vi "Reinitial Parameter After Test.vi"(8 "error in (no error)":errorcluster, 11 "main ref":T1) -> (0 "error out":errorcluster)   [LabVIEW 2025]
uses:
  controls/LAB-IQ UI Data.ctl
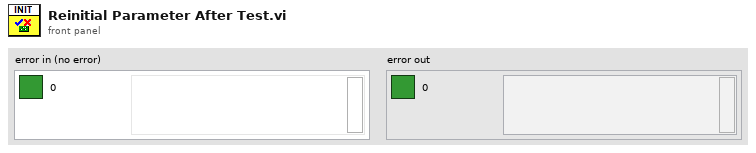
[diagram p1: front panel]
types:
  T1 = typedef "LAB-IQ UI Data.ctl" = cluster{"Main Home Screen":cluster{"GUI":refnum<vi>, "Platform Settings":refnum<vi>, "Configure":refnum<vi>, "Home":refnum<vi>, "EXIT":refnum<vi>, "service 2":refnum<vi>, "MainPage":refnum<vi>, "Analysis":refnum<vi>}, "Platform Settings":cluster{"mm/s  Surge":refnum<vi>, "Update Surge Speed":refnum<vi>, "Drive Error":refnum<vi>, "Disable Axis Jog Soft Limits":refnum<vi>, "mm/s  Sway":refnum<vi>, "Sway and Surge COM Status":refnum<vi>, "Heave COM Status":refnum<vi>, "Enable Platform":refnum<vi>, "Surge Forward Main":refnum<vi>, "Sway Right Main":refnum<vi>, "Sway Left Main":refnum<vi>, "Heave Down Main":refnum<vi>, "Heave Up main":refnum<vi>, "Update Sway Speed":refnum<vi>, "Update Heave Speed":refnum<vi>, "mm/s Heave":refnum<vi>, "mm/sec":refnum<vi>, "mm":refnum<vi>, "Surge Backward Main":refnum<vi>}, "Analysis Screen":cluster{"Analysis Home":refnum<vi>, "Surface Analysis":refnum<vi>, "Imaging":refnum<vi>, "Image Analysis":refnum<vi>, "Post Analysis":refnum<vi>}, "Config Screen":cluster{"Select Load Head":refnum<vi>, "Notes :":refnum<vi>, "FILE":refnum<vi>, "Sample ID :":refnum<vi>, "Operator ID :":refnum<vi>, "Operator Name :":refnum<vi>, "Auto":refnum<vi>}, "Motion Module":cluster{"zNL":refnum<vi>, "NL disp":refnum<vi>, "Rotary Tab":refnum<vi>, "Motion Direction:  3":refnum<vi>, "E.Velocity 2":refnum<vi>, "e.v/ssr 2":refnum<vi>, "Enter Fixed E.Velocity 2":refnum<vi>, "Enter Final SRR 2":refnum<vi>, "Enter initial SRR 2":refnum<vi>, "Enter Fixed SRR 2":refnum<vi>, "Enter the Final E.Velocity (m/s) 2":refnum<vi>, "Enter initial E.Velocity (m/s) 2":refnum<vi>, "Final Speed (RPM) 3":refnum<vi>, "Initial Speed (RPM) 2":refnum<vi>, "Enter the Final Velocity (m/s) 3":refnum<vi>, "Enter initial Velocity (m/s)  3":refnum<vi>, "Ramp Up 2":refnum<vi>, "TEST SELECTION":refnum<vi>, "SPEED SELECTION : ":refnum<vi>, "Angular Oscillation Set":refnum<vi>, "Traction":refnum<vi>, "Step Speed":refnum<vi>, "StepTable For Load-Speed":refnum<vi>, "StepTable For Speed":refnum<vi>, "Surge Forward MM":refnum<vi>, "Surge Backward MM":refnum<vi>, "M3 Image":refnum<vi>, "String 39":refnum<vi>, "Sway Left MM":refnum<vi>, "Sway Right MM":refnum<vi>, "Disable Axis Jog Soft Limits":refnum<vi>, "mm":refnum<vi>, "Heave Down MM":refnum<vi>, "Heave Up MM":refnum<vi>, "Wear Track Diameter (mm)":refnum<vi>, "Set WTD":refnum<vi>, "HomeScratch":refnum<vi>, "HomeRot":refnum<vi>, "PlaceModule":refnum<vi>, "Enter the Angle (Deg)":refnum<vi>, "Enter the Frequency (Hz)":refnum<vi>, "Motion Mode:":refnum<vi>, "LR Sway":refnum<vi>, "Rot Hor":refnum<vi>, "Scratch":refnum<vi>, "LR Cam":refnum<vi>, "MMBack":refnum<vi>, "MMNext":refnum<vi>, "Rot Ver":refnum<vi>, "Rotary Module Selection":refnum<vi>, "calculate rotary":refnum<vi>, "SPEED SELECTION : rotary":refnum<vi>, "Import 2":refnum<vi>, "Save 2":refnum<vi>, "File Path :  2":refnum<vi>, "String 45":refnum<vi>, "StepTable For Speed 3":refnum<vi>, "Enter the Speed(mm/sec)":refnum<vi>, "Enter the Speed(RPM)":refnum<vi>, "Enter Scratch Speed (mm/s):":refnum<vi>, "SwaySpeed Set":refnum<vi>, "Scartch Offset":refnum<vi>, "Motion type:":refnum<vi>, "HomeScratch 2":refnum<vi>, "Enter Scratch length (mm):":refnum<vi>, "Wear Track Diameter":refnum<vi>, "Rotary Speed Exced":refnum<vi>, "Scratch Mode":refnum<vi>, "No of Scratch":refnum<vi>}, "Environmental control":cluster{"Humidity  Status  3":refnum<vi>, "Low Temp  Status  2":refnum<vi>, "TK4 status 2":refnum<vi>, "Stage Temperature":refnum<vi>, "Sample Temperature":refnum<vi>, "Humidity (Amb)":refnum<vi>, "Clear List":refnum<vi>, "Add to list":refnum<vi>, "Wear":refnum<vi>, "Vibration":refnum<vi>, "Humidity (Chamber)":refnum<vi>, "Temperature (Chamber)":refnum<vi>, "ECR ":refnum<vi>, "Temperature (Amb)":refnum<vi>, "Microphone":refnum<vi>, "Acoustic Emission 3":refnum<vi>, "SNext":refnum<vi>, "APBack":refnum<vi>, "Enter the Temperature (°C):":refnum<vi>, "Enter the Stage \nTemperature (°C):":refnum<vi>, "Enter the Humidity (%Rh):":refnum<vi>, "Low Temp":refnum<vi>, "High Temp":refnum<vi>, "Humidity":refnum<vi>, "Sensors Picked":refnum<vi>}, "About Screen":cluster{"Password":refnum<vi>, "Home Service":refnum<vi>, "Advanced Setting":refnum<vi>, "About Tab":refnum<vi>, "ECR Port:":refnum<vi>, "Ramp Port:":refnum<vi>, "Installation/Replacement completed":refnum<vi>, "Loahead":refnum<vi>, "Heave and Surge COM Port:":refnum<vi>, "Sway COM Port:":refnum<vi>, "Temp Modbus:":refnum<vi>, "Humidity Port:":refnum<vi>, "Edit Gain Constants":refnum<vi>, "Save Gain Constants":refnum<vi>}, "Main Screen":cluster{"Main Screen Tab":refnum<vi>, "Angle and Frequency":refnum<vi>, "Stroke (mm)":refnum<vi>, "Angle (Deg)":refnum<vi>, "Main Speed Tab":refnum<vi>, "MTM MOTOR DISPLAY":refnum<vi>, "Disc Speed (m/sec)":refnum<vi>, "Ball Speed (m/sec)":refnum<vi>, "Disc Speed (RPM)":refnum<vi>, "Ball Speed (RPM)":refnum<vi>, "SPEED TAB":refnum<vi>, "Speed (m/sec)":refnum<vi>, "Set Speed (m/sec)":refnum<vi>, "Speed (RPM)":refnum<vi>, "Set Speed":refnum<vi>, "Time Tab":refnum<vi>, "Time ( HH:MM:SS ) 2":refnum<vi>, "Test Duration":refnum<vi>, "Test Duration 4":refnum<vi>, "TEST CYCLE":refnum<vi>, "TOTAL CYCLES":refnum<vi>, "Set Load (N)":refnum<vi>, "Temp Tabs":refnum<vi>, "Heater":refnum<vi>, "TK4 status":refnum<vi>, "ChamberTemp":refnum<vi>, "SetTmp":refnum<vi>, "Controller  Status":refnum<vi>, "ChamberTemp 2":refnum<vi>, "SetTmp 2":refnum<vi>, "Controller  Status 2":refnum<vi>, "ChamberTemp 3":refnum<vi>, "SetTmp 3":refnum<vi>, "Cooling":refnum<vi>, "Load Communication":refnum<vi>, "Ambient \nTemperature":refnum<vi>, "HumCOMStatus":refnum<vi>, "Ambient\n Humidity":refnum<vi>, "Freq (Hz)":refnum<vi>, "Load En":refnum<vi>, "NLt":refnum<vi>, "zNL 2":refnum<vi>, "Humidity On":refnum<vi>, "humidity disp":refnum<vi>, "Set Humidity":refnum<vi>, "NL disp 2":refnum<vi>, "Humidity On 2":refnum<vi>, "humidity disp 2":refnum<vi>, "Set Humidity 2":refnum<vi>, "NL disp 3":refnum<vi>, "AppLoadSeq scratch":refnum<vi>, "Stop Scratch":refnum<vi>, "ClrLog":refnum<vi>, "Trip Log":refnum<vi>, "STOP":refnum<vi>, "Start Test":refnum<vi>, "Test status":refnum<vi>, "AR Led":refnum<vi>, "Data":refnum<vi>, "Health":refnum<vi>, "Sway COM Status":refnum<vi>, "Heave COM Status":refnum<vi>, "Grp Tab":refnum<vi>, "Sub Graph":refnum<vi>, "SD (mm)":refnum<vi>, "Siliding distance Reset Graph":refnum<vi>, "SDGp":refnum<vi>, "Humidity Reset Graph":refnum<vi>, "HumrGp":refnum<vi>, "Acoustic Emission (mV)":refnum<vi>, "Aqucostic Reset Graph":refnum<vi>, "gACQUOS":refnum<vi>, "ECR RESET":refnum<vi>, "ECR":refnum<vi>, "Temperature Reset":refnum<vi>, "Acoustic Emission (mV) 2":refnum<vi>, "Aqucostic Reset Graph 2":refnum<vi>, "gACQUOS 2":refnum<vi>, "ECR RESET 2":refnum<vi>, "ECR 2":refnum<vi>, "Temperature Reset 2":refnum<vi>, "Temperature (deg c)":refnum<vi>, "Speed Reset Graph":refnum<vi>, "Speed Tab":refnum<vi>, "MTM DISC  SPEED":refnum<vi>, "MTM BALL SPEED":refnum<vi>, "speed mm/sec":refnum<vi>, "Hymidity":refnum<vi>, "Humidity Disable trip":refnum<vi>, "CoF Trip  2":refnum<vi>, "Depth Trip":refnum<vi>, "Weart Deapth":refnum<vi>, "Depth Reset Graph":refnum<vi>, "Weart":refnum<vi>, "Depthz":refnum<vi>, "Depth (µm)":refnum<vi>, "WearGp":refnum<vi>, "NL Trip 2":refnum<vi>, "Load pid":refnum<vi>, "Load Disable Trip":refnum<vi>, "Load Reset Graph":refnum<vi>, "NL Display 4":refnum<vi>, "Main Chart 3":refnum<vi>, "BACK":refnum<vi>, "Depth Trip 2":refnum<vi>, "COF TRIP ":refnum<vi>, "Friction Force (N)":refnum<vi>, "FF Reset Graph":refnum<vi>, "FF Disable Trip":refnum<vi>, "FF TRIP":refnum<vi>, "COF Disable Trip":refnum<vi>, "COF Reset Graph":refnum<vi>, "Start Test Temp":refnum<vi>, "zFF":refnum<vi>, "Friction Force (N) Graph":refnum<vi>, "Coefficient of Friction":refnum<vi>, "Scratch Start Test":refnum<vi>, "FF Tab":refnum<vi>, "Cyclic Friction Force (N)":refnum<vi>, "CZ FF":refnum<vi>, "Cyclic Friction Force (N) Graph":refnum<vi>, "Cyclic Coefficient of Friction":refnum<vi>, "Cyclic FF TRIP":refnum<vi>, "Cyclic FF Disable Trip":refnum<vi>, "cyclic COF Disable Trip":refnum<vi>, "cyclic COF TRIP":refnum<vi>, "cyclic COF Reset Graph":refnum<vi>, "Cyclic FF Reset Graph":refnum<vi>, "Test Trip":refnum<vi>, "Multi Scratch Pass":refnum<vi>, "Scratch Start Recording":refnum<vi>}, "Loading":cluster{"Indentation":refnum<vi>, "Reference Sample":refnum<vi>, "Load Cell Communication Slide":refnum<vi>, "com 3":refnum<vi>, "com":refnum<vi>, "DecaForce COM Status":refnum<vi>, "Update":refnum<vi>, "Clear 3":refnum<vi>, "seq":refnum<vi>, "Stribeck table":refnum<vi>, "Stribeck Table  For loading":refnum<vi>, "Loading Mode":refnum<vi>, "Enter the Final Load (N)":refnum<vi>, "Enter the CoF Trip":refnum<vi>, "Enter the Friction Force Trip":refnum<vi>, "Enter the Normal load Trip":refnum<vi>, "Enter the Load  (N)":refnum<vi>, "KiloForce":refnum<vi>, "DecaForce ":refnum<vi>, "MicroForce":refnum<vi>, "LHBack":refnum<vi>, "LHNext":refnum<vi>, "Enter the Loading Rate (N/min)":refnum<vi>, "Message":refnum<vi>, "Warning 2":refnum<vi>, "SSP 0.75":refnum<vi>, "SSP 0.5":refnum<vi>, "SSP 0.3":refnum<vi>, "Warning":refnum<vi>, "gui GIF":refnum<vi>, "Communication is established":refnum<vi>, "AppLoad 4":refnum<vi>, "Multipoint":refnum<vi>, "Load Selection":refnum<vi>}, "PID":cluster{"Ramp MulFac":refnum<vi>, "pulses LoadDiffRamp(2..10)":refnum<vi>, "PulseControlRamp(diff<=3N)":refnum<vi>, "SetLoadDeadband(%) Load(0-10N)":refnum<vi>, "PID gains out delay (microForce)":refnum<vi>, "Ramp":refnum<vi>, "Gain 2":refnum<vi>, "pulses LoadDiff(2..10)":refnum<vi>, "pulses LoadDiff(11..50)":refnum<vi>, "PulseControl(diff<=3N)":refnum<vi>, "SetLoadDeadband(%)  2":refnum<vi>, "Dummy Run":refnum<vi>, "Vertical load (N)":refnum<vi>, "AutoTune":refnum<vi>, "Offset 3 ":refnum<vi>, "apply load":refnum<vi>, "Offset  3":refnum<vi>, "apply load 2":refnum<vi>, "Enter ByPass Load":refnum<vi>, "reinit 3":refnum<vi>, "output range delay":refnum<vi>, "PID gains out delay":refnum<vi>, "Bypass Load":refnum<vi>, "pulsesSent":refnum<vi>, "pulses ":refnum<vi>, "actpid":refnum<vi>, "gFF Rot":refnum<vi>, "pulses LoadDiff(21..1000)":refnum<vi>, "Delay":refnum<vi>, "deadband":refnum<vi>}, "Config Parameters":cluster{"Tab Control 3":refnum<vi>, "Tab Control 19":refnum<vi>, "SAMPLES":refnum<vi>, "Re-initilaize":refnum<vi>, "Filter ON/OFF":refnum<vi>, "TracHomeSurgeOffsetCounts 10MM":refnum<vi>, "TracHomeSwayOffsetCounts 10MM":refnum<vi>, "Acoustic Emission:":refnum<vi>, "Apply Filter (FF)":refnum<vi>, "Filter% 2":refnum<vi>, "Apply Filter (Load)":refnum<vi>, "Filter% ":refnum<vi>, "Sway distance (mm)":refnum<vi>, "Surge distance (mm)":refnum<vi>, "DataSavingLoopDelay(ms)":refnum<vi>, "SAVE 2":refnum<vi>, "Enter Distance":refnum<vi>, "Sway Counts:":refnum<vi>, "Distance (mm): 3":refnum<vi>, "Surge Counts:":refnum<vi>, "Distance (mm): 2":refnum<vi>, "Distance (mm):":refnum<vi>, "Heave Counts:":refnum<vi>, "LRMHomeSurgeOffsetCounts":refnum<vi>, "LRMHomeSwayOffsetCounts":refnum<vi>, "TracHomeSurgeOffsetCounts 20MM":refnum<vi>, "TracHomeSwayOffsetCounts 20MM":refnum<vi>, "RotHomeSwayOffsetCounts":refnum<vi>, "RotHomeSurgeOffsetCounts":refnum<vi>, "Heave distance":refnum<vi>, "Zmm":refnum<vi>, "Heave Pulses/mm":refnum<vi>, "Surge Pulses/mm":refnum<vi>, "Sway Pulses/mm":refnum<vi>, "Heave Pitch":refnum<vi>, "Surge Pitch":refnum<vi>, "Sway Pitch":refnum<vi>, "Heave PPR":refnum<vi>, "Surge PPR":refnum<vi>, "Sway PPR":refnum<vi>, "Tab Control 5":refnum<vi>, "Tab Control 14":refnum<vi>, "Tab Control 26":refnum<vi>, "AE":refnum<vi>, "Heave Loop Delay":refnum<vi>, "Heave PID Speed":refnum<vi>, "Surge Jog Speed":refnum<vi>, "Heave Jog Speed":refnum<vi>, "Sway Loop Delay":refnum<vi>, "Sway PID Speed":refnum<vi>, "Sway Jog Speed":refnum<vi>, "DEPTH TRIP VALUE":refnum<vi>, "LOAD TRIP VALUE":refnum<vi>, "DEPTH TRIP   ENABLE":refnum<vi>, "LOAD TRIP  ENABLE":refnum<vi>, "CYCLIC FF TRIP VALUE":refnum<vi>, "FF TRIP VALUE":refnum<vi>, "CYCLIC CoF TRIP VALUE":refnum<vi>, "COF TRIP VALUE":refnum<vi>, "CYCLIC COF TRIP  ENABLE":refnum<vi>, "CYCLIC FF TRIP  ENABLE":refnum<vi>, "FF TRIP  ENABLE":refnum<vi>, "COF TRIP  ENABLE":refnum<vi>}, "Loading Com Port":cluster{"ClearAll":refnum<vi>, "Mz(Nm)":refnum<vi>, "My(Nm)":refnum<vi>, "Mx(Nm)":refnum<vi>, "Save Dwell":refnum<vi>, "Mx ":refnum<vi>, "My ":refnum<vi>, "Mz":refnum<vi>, "Fx(N)":refnum<vi>, "Fy(N)":refnum<vi>, "Fz(N)":refnum<vi>, "ZeroAll":refnum<vi>, "Acq Delay (ms)":refnum<vi>, "Burst Delay (ms)":refnum<vi>, "model":refnum<vi>, "SN":refnum<vi>, "FFx(N)":refnum<vi>, "Sensor IP":refnum<vi>, "Port":refnum<vi>, "FFy(N)":refnum<vi>, "Load(N)":refnum<vi>, "delete Handle":refnum<vi>, "Create Handle":refnum<vi>, "ft_data":refnum<vi>, "ft_range":refnum<vi>, "ft_data 2":refnum<vi>, "stop 6":refnum<vi>, "running_flag":refnum<vi>, "ft_udp_handle":refnum<vi>, "get-data-return":refnum<vi>, "get-range-return":refnum<vi>, "zero-return":refnum<vi>, "filter-return":refnum<vi>, "initial-return":refnum<vi>, "deleteHandle-result":refnum<vi>, "Load Cell Temp":refnum<vi>}, "Heave AND Surge":cluster{"SURGE POSE":refnum<vi>, "error out Read":refnum<vi>, "HEAVE POSE":refnum<vi>, "State":refnum<vi>, "Homed":refnum<vi>, "Sequence ID":refnum<vi>, "error out Write":refnum<vi>, "faultCode":refnum<vi>, "Ack ID":refnum<vi>, "SPEED":refnum<vi>, "Distance":refnum<vi>, "Mode Command":refnum<vi>, "Heave and Surge Read":refnum<vi>, "Read Heave Temp":refnum<vi>, "Spare 15":refnum<vi>, "Spare 14":refnum<vi>, "Spare 13":refnum<vi>, "Spare 12":refnum<vi>, "Spare 11":refnum<vi>, "Spare 10":refnum<vi>, "Spare 9":refnum<vi>, "Spare 8":refnum<vi>, "Spare 7":refnum<vi>, "Spare 6":refnum<vi>, "Spare 5":refnum<vi>, "Spare 4":refnum<vi>, "Spare 2":refnum<vi>, "Spare 1":refnum<vi>, "Node Id":refnum<vi>, "Spare 3":refnum<vi>, "SPARE 4":refnum<vi>, "SPARE 3":refnum<vi>, "SPARE 2":refnum<vi>, "SPARE 1":refnum<vi>, "fwMajor":refnum<vi>, "fwMinor":refnum<vi>, "Manual Write":refnum<vi>, "Heave and Surge Write":refnum<vi>}, "New PID LOGIC":cluster{"Fine Tune Zone":refnum<vi>, "PID SDelay":refnum<vi>, "Max_pos_limit":refnum<vi>, "Min_pos_limit":refnum<vi>, "i_limit":refnum<vi>, "pct_scale":refnum<vi>, "Deadband":refnum<vi>, "Kd":refnum<vi>, "Ki":refnum<vi>, "Kp":refnum<vi>, "Current Position":refnum<vi>, "Set Load":refnum<vi>, "Current Load":refnum<vi>, "Pulse delta":refnum<vi>, "Init Step":refnum<vi>, "Max Step Linit":refnum<vi>}, "SWAY ":cluster{"fwMajor":refnum<vi>, "Homed":refnum<vi>, "Rotary POSE":refnum<vi>, "State":refnum<vi>, "SWAY POSE":refnum<vi>, "Ack ID":refnum<vi>, "faultCode":refnum<vi>, "Node Id":refnum<vi>, "fwMinor":refnum<vi>, "Spare 6":refnum<vi>, "Spare 5":refnum<vi>, "Spare 4":refnum<vi>, "Spare 3":refnum<vi>, "Spare 2":refnum<vi>, "Spare 1":refnum<vi>, "Spare 7":refnum<vi>, "SPARE  5":refnum<vi>, "error out Write  SWAY ":refnum<vi>, "error out Read SWAY ":refnum<vi>, "Manual Write SWAY ":refnum<vi>, "SWAY WRITE":refnum<vi>, "SPARE  4":refnum<vi>, "SPARE  3":refnum<vi>, "SPARE 2":refnum<vi>, "SPARE 1":refnum<vi>, "Spare 15":refnum<vi>, "Spare 14":refnum<vi>, "Spare 13":refnum<vi>, "Spare 12":refnum<vi>, "Spare 11":refnum<vi>, "Spare 9":refnum<vi>, "Spare 8":refnum<vi>, "SPEED":refnum<vi>, "Distance":refnum<vi>, "Mode Command":refnum<vi>, "Sequence ID":refnum<vi>, "SWAY READ":refnum<vi>, "Spare 10":refnum<vi>, "Read SWAY Temp":refnum<vi>}, "Analysis Screen":cluster{"Analysis Home":refnum<vi>, "Refresh 2":refnum<vi>, "MEAN 4":refnum<vi>, "SD 4":refnum<vi>, "VARIANCE 4":refnum<vi>, "MEAN  3":refnum<vi>, "SD  3":refnum<vi>, "VARIANCE  3":refnum<vi>, "MEAN 2":refnum<vi>, "SD  2":refnum<vi>, "VARIANCE 2":refnum<vi>, "MEAN":refnum<vi>, "SD":refnum<vi>, "VARIANCE":refnum<vi>, "File 4 Discription":refnum<vi>, "OPEN 4":refnum<vi>, "File Name 4":refnum<vi>, "OPEN 3":refnum<vi>, "File 3 Discription":refnum<vi>, "File Name 3":refnum<vi>, "Y-AXIS":refnum<vi>, "X-AXIS":refnum<vi>, "XY Graph":refnum<vi>, "File Name 2":refnum<vi>, "File Name 1":refnum<vi>, "OPEN 2":refnum<vi>, "OPEN 1":refnum<vi>, "File 1 Discription ":refnum<vi>, "File 2 Discription":refnum<vi>, "Export":refnum<vi>, "File Format":refnum<vi>}}
  T2 = enum8{"Enabled", "Disabled", "Disabled and Grayed Out"}
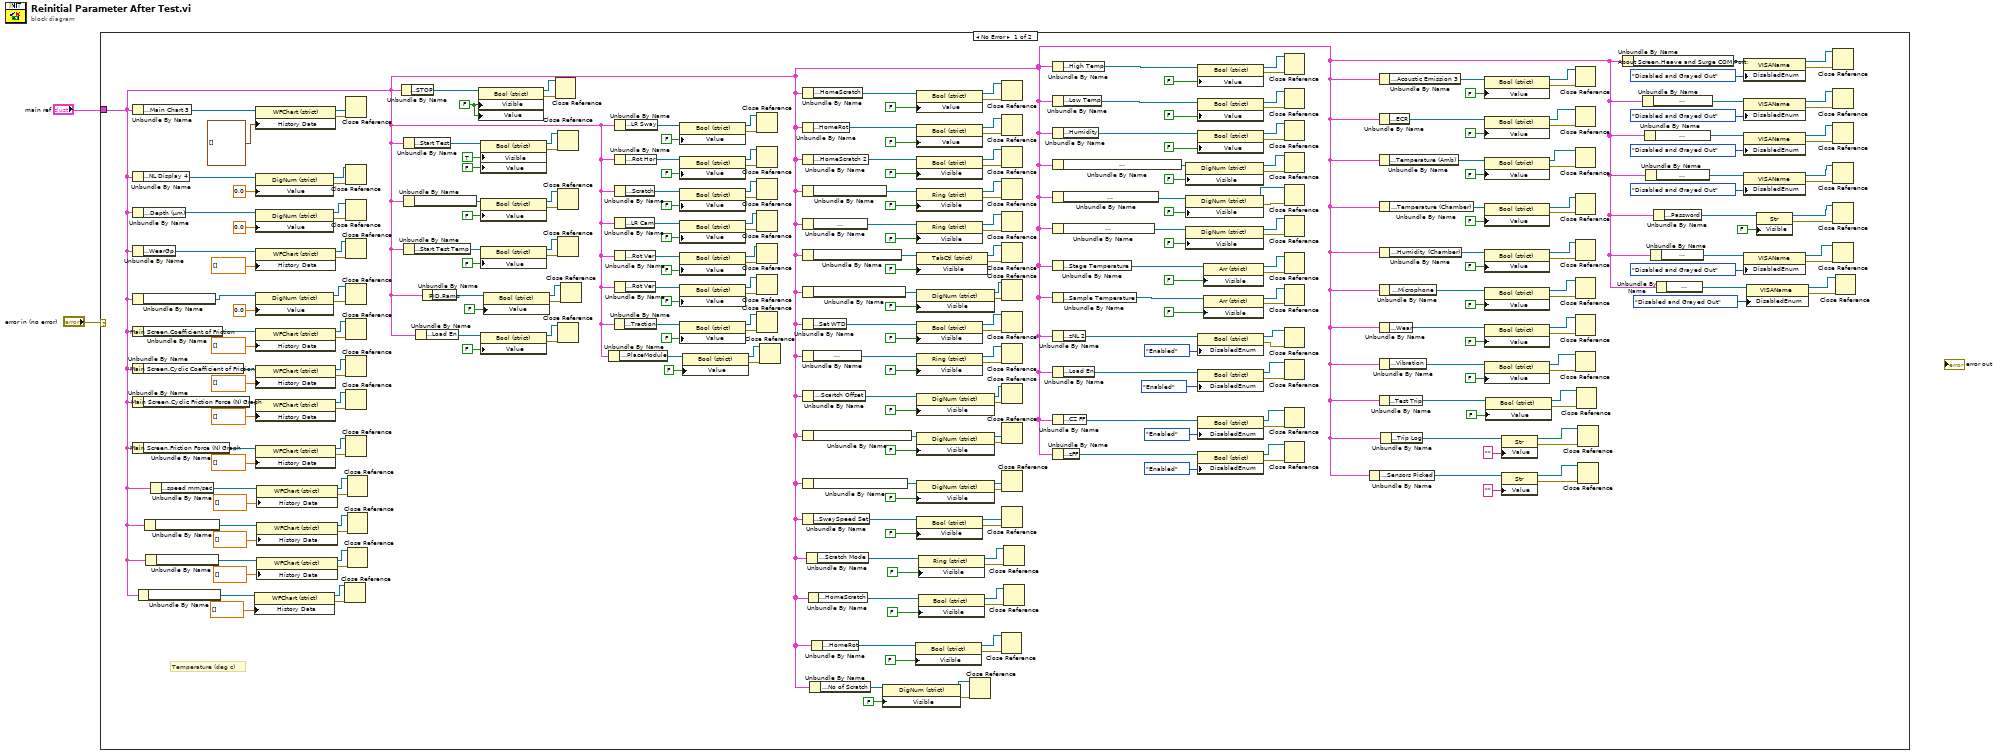
[diagram p0: block diagram]
diagram:
  n1 = case shown="No Error" "error in (no error)" {
    tunnel: "main ref" -> [w3 _]
    frame No Error {
      w233 = FALSE ("Visible")
      # "Temperature (deg c)"
      n2 = Unbundle By Name(w3) -> ("Main Screen.Main Chart 3"=w298:refnum<vi>)
      n3 = Unbundle By Name(w3) -> ("Main Screen.NL Display 4"=w296:refnum<vi>)
      n4 = Unbundle By Name(w3) -> ("Main Screen.Depth (µm)"=w291:refnum<vi>)
      n5 = Unbundle By Name(w3) -> ("Main Screen.WearGp"=w288:refnum<vi>)
      n6 = Unbundle By Name(w3) -> ("Main Screen.Time ( HH:MM:SS ) 2"=w284:refnum<vi>)
      n7 = Unbundle By Name(w3) -> ("Main Screen.Coefficient of Friction"=w281:refnum<vi>)
      n8 = Unbundle By Name(w3) -> ("Main Screen.Cyclic Coefficient of Friction"=w273:refnum<vi>)
      n9 = Unbundle By Name(w3) -> ("Main Screen.Cyclic Friction Force (N) Graph"=w277:refnum<vi>)
      n10 = Unbundle By Name(w3) -> ("Main Screen.Friction Force (N) Graph"=w269:refnum<vi>)
      n11 = Unbundle By Name(w3) -> ("Main Screen.Temperature (deg c)"=w252:refnum<vi>)
      n12 = Unbundle By Name(w3) -> ("Main Screen.MTM DISC  SPEED"=w259:refnum<vi>)
      n13 = Unbundle By Name(w3) -> ("Main Screen.MTM BALL SPEED"=w254:refnum<vi>)
      n14 = Unbundle By Name(w3) -> ("Main Screen.speed mm/sec"=w262:refnum<vi>)
      n15 = property class="WFChart (strict)"(reference=w252, "History Data"=dbl[] []) -> (reference out=w249:refnum<vi>, error out=w251:errorcluster)  [unwired: 1 in]
      n16 = property class="WFChart (strict)"(reference=w298, "History Data"=cluster{dbl, "NL disp":dbl, dbl}[] []) -> (reference out=w300:refnum<vi>, error out=w299:errorcluster)  [unwired: 1 in]
      n17 = property class="DigNum (strict)"(reference=w296, "Value"=0.0) -> (reference out=w294:refnum<vi>, error out=w295:errorcluster)  [unwired: 1 in]
      n18 = property class="DigNum (strict)"(reference=w291, "Value"=0.0) -> (reference out=w292:refnum<vi>, error out=w290:errorcluster)  [unwired: 1 in]
      n19 = property class="WFChart (strict)"(reference=w288, "History Data"=dbl[] []) -> (reference out=w286:refnum<vi>, error out=w287:errorcluster)  [unwired: 1 in]
      n20 = property class="DigNum (strict)"(reference=w284, "Value"=0.0) -> (reference out=w265:refnum<vi>, error out=w285:errorcluster)  [unwired: 1 in]
      n21 = property class="WFChart (strict)"(reference=w281, "History Data"=dbl[] []) -> (reference out=w282:refnum<vi>, error out=w280:errorcluster)  [unwired: 1 in]
      n22 = property class="WFChart (strict)"(reference=w273, "History Data"=dbl[] []) -> (reference out=w272:refnum<vi>, error out=w274:errorcluster)  [unwired: 1 in]
      n23 = property class="WFChart (strict)"(reference=w277, "History Data"=dbl[] []) -> (reference out=w275:refnum<vi>, error out=w276:errorcluster)  [unwired: 1 in]
      n24 = property class="WFChart (strict)"(reference=w269, "History Data"=dbl[] []) -> (reference out=w267:refnum<vi>, error out=w268:errorcluster)  [unwired: 1 in]
      n25 = property class="WFChart (strict)"(reference=w262, "History Data"=dbl[] []) -> (reference out=w261:refnum<vi>, error out=w263:errorcluster)  [unwired: 1 in]
      n26 = property class="WFChart (strict)"(reference=w259, "History Data"=dbl[] []) -> (reference out=w260:refnum<vi>, error out=w258:errorcluster)  [unwired: 1 in]
      n27 = property class="WFChart (strict)"(reference=w254, "History Data"=dbl[] []) -> (reference out=w253:refnum<vi>, error out=w255:errorcluster)  [unwired: 1 in]
      n28 = Close Reference(reference=w249, error in (no error)=w251) -> ()  [unwired: 1 out]
      n29 = Close Reference(reference=w300, error in (no error)=w299) -> ()  [unwired: 1 out]
      n30 = Close Reference(reference=w294, error in (no error)=w295) -> ()  [unwired: 1 out]
      n31 = Close Reference(reference=w292, error in (no error)=w290) -> ()  [unwired: 1 out]
      n32 = Close Reference(reference=w286, error in (no error)=w287) -> ()  [unwired: 1 out]
      n33 = Close Reference(reference=w265, error in (no error)=w285) -> ()  [unwired: 1 out]
      n34 = Close Reference(reference=w282, error in (no error)=w280) -> ()  [unwired: 1 out]
      n35 = Close Reference(reference=w272, error in (no error)=w274) -> ()  [unwired: 1 out]
      n36 = Close Reference(reference=w275, error in (no error)=w276) -> ()  [unwired: 1 out]
      n37 = Close Reference(reference=w267, error in (no error)=w268) -> ()  [unwired: 1 out]
      n38 = Close Reference(reference=w261, error in (no error)=w263) -> ()  [unwired: 1 out]
      n39 = Close Reference(reference=w260, error in (no error)=w258) -> ()  [unwired: 1 out]
      n40 = Close Reference(reference=w253, error in (no error)=w255) -> ()  [unwired: 1 out]
      n41 = Unbundle By Name(w3) -> ("Main Screen.STOP"=w239:refnum<vi>)
      n42 = Unbundle By Name(w3) -> ("Main Screen.Start Test"=w237:refnum<vi>)
      n43 = Unbundle By Name(w3) -> ("Main Screen.Scratch Start Test"=w245:refnum<vi>)
      n44 = Unbundle By Name(w3) -> ("Main Screen.Start Test Temp"=w246:refnum<vi>)
      n45 = Unbundle By Name(w3) -> ("Main Screen.Load En"=w225:refnum<vi>)
      n46 = Unbundle By Name(w3) -> ("PID.Ramp"=w230:refnum<vi>)
      n47 = property class="Bool (strict)"(reference=w239, "Visible"=w233, "Value"=w233) -> (reference out=w234:refnum<vi>, error out=w240:errorcluster)  [unwired: 1 in]
      n48 = property class="Bool (strict)"(reference=w237, "Visible"=TRUE, "Value"=FALSE) -> (reference out=w235:refnum<vi>, error out=w236:errorcluster)  [unwired: 1 in]
      n49 = property class="Bool (strict)"(reference=w245, "Value"=FALSE) -> (reference out=w243:refnum<vi>, error out=w244:errorcluster)  [unwired: 1 in]
      n50 = property class="Bool (strict)"(reference=w246, "Value"=FALSE) -> (reference out=w248:refnum<vi>, error out=w247:errorcluster)  [unwired: 1 in]
      n51 = property class="Bool (strict)"(reference=w225, "Value"=FALSE) -> (reference out=w227:refnum<vi>, error out=w226:errorcluster)  [unwired: 1 in]
      n52 = property class="Bool (strict)"(reference=w230, "Value"=FALSE) -> (reference out=w228:refnum<vi>, error out=w229:errorcluster)  [unwired: 1 in]
      n53 = Close Reference(reference=w234, error in (no error)=w240) -> ()  [unwired: 1 out]
      n54 = Close Reference(reference=w235, error in (no error)=w236) -> ()  [unwired: 1 out]
      n55 = Close Reference(reference=w243, error in (no error)=w244) -> ()  [unwired: 1 out]
      n56 = Close Reference(reference=w248, error in (no error)=w247) -> ()  [unwired: 1 out]
      n57 = Close Reference(reference=w227, error in (no error)=w226) -> ()  [unwired: 1 out]
      n58 = Close Reference(reference=w228, error in (no error)=w229) -> ()  [unwired: 1 out]
      n59 = Unbundle By Name(w3) -> ("Motion Module.PlaceModule"=w194:refnum<vi>)
      n60 = Unbundle By Name(w3) -> ("Motion Module.Traction"=w198:refnum<vi>)
      n61 = Unbundle By Name(w3) -> ("Motion Module.LR Sway"=w221:refnum<vi>)
      n62 = Unbundle By Name(w3) -> ("Motion Module.Rot Hor"=w218:refnum<vi>)
      n63 = Unbundle By Name(w3) -> ("Motion Module.Scratch"=w214:refnum<vi>)
      n64 = Unbundle By Name(w3) -> ("Motion Module.LR Cam"=w209:refnum<vi>)
      n65 = Unbundle By Name(w3) -> ("Motion Module.Rot Ver"=w206:refnum<vi>)
      n66 = Unbundle By Name(w3) -> ("Motion Module.Rot Ver"=w202:refnum<vi>)
      n67 = property class="Bool (strict)"(reference=w221, "Value"=FALSE) -> (reference out=w223:refnum<vi>, error out=w222:errorcluster)  [unwired: 1 in]
      n68 = property class="Bool (strict)"(reference=w218, "Value"=FALSE) -> (reference out=w216:refnum<vi>, error out=w217:errorcluster)  [unwired: 1 in]
      n69 = property class="Bool (strict)"(reference=w214, "Value"=FALSE) -> (reference out=w212:refnum<vi>, error out=w215:errorcluster)  [unwired: 1 in]
      n70 = property class="Bool (strict)"(reference=w209, "Value"=FALSE) -> (reference out=w211:refnum<vi>, error out=w208:errorcluster)  [unwired: 1 in]
      n71 = property class="Bool (strict)"(reference=w206, "Value"=FALSE) -> (reference out=w204:refnum<vi>, error out=w207:errorcluster)  [unwired: 1 in]
      n72 = property class="Bool (strict)"(reference=w202, "Value"=FALSE) -> (reference out=w200:refnum<vi>, error out=w201:errorcluster)  [unwired: 1 in]
      n73 = property class="Bool (strict)"(reference=w198, "Value"=FALSE) -> (reference out=w196:refnum<vi>, error out=w197:errorcluster)  [unwired: 1 in]
      n74 = property class="Bool (strict)"(reference=w194, "Value"=FALSE) -> (reference out=w192:refnum<vi>, error out=w193:errorcluster)  [unwired: 1 in]
      n75 = Close Reference(reference=w223, error in (no error)=w222) -> ()  [unwired: 1 out]
      n76 = Close Reference(reference=w216, error in (no error)=w217) -> ()  [unwired: 1 out]
      n77 = Close Reference(reference=w212, error in (no error)=w215) -> ()  [unwired: 1 out]
      n78 = Close Reference(reference=w211, error in (no error)=w208) -> ()  [unwired: 1 out]
      n79 = Close Reference(reference=w204, error in (no error)=w207) -> ()  [unwired: 1 out]
      n80 = Close Reference(reference=w200, error in (no error)=w201) -> ()  [unwired: 1 out]
      n81 = Close Reference(reference=w196, error in (no error)=w197) -> ()  [unwired: 1 out]
      n82 = Close Reference(reference=w192, error in (no error)=w193) -> ()  [unwired: 1 out]
      n83 = Unbundle By Name(w3) -> ("Motion Module.HomeScratch"=w162:refnum<vi>)
      n84 = Unbundle By Name(w3) -> ("Motion Module.HomeRot"=w165:refnum<vi>)
      n85 = Unbundle By Name(w3) -> ("Motion Module.HomeScratch 2"=w169:refnum<vi>)
      n86 = Unbundle By Name(w3) -> ("Motion Module.Motion Direction:  3"=w174:refnum<vi>)
      n87 = Unbundle By Name(w3) -> ("Motion Module.Motion Mode:"=w177:refnum<vi>)
      n88 = Unbundle By Name(w3) -> ("Motion Module.Rotary Module Selection"=w181:refnum<vi>)
      n89 = Unbundle By Name(w3) -> ("Motion Module.Wear Track Diameter (mm)"=w185:refnum<vi>)
      n90 = Unbundle By Name(w3) -> ("Motion Module.Set WTD"=w189:refnum<vi>)
      n91 = Unbundle By Name(w3) -> ("Motion Module.Motion type:"=w158:refnum<vi>)
      n92 = Unbundle By Name(w3) -> ("Motion Module.Scartch Offset"=w155:refnum<vi>)
      n93 = Unbundle By Name(w3) -> ("Motion Module.Enter Scratch Speed (mm/s):"=w150:refnum<vi>)
      n94 = Unbundle By Name(w3) -> ("Motion Module.Enter Scratch length (mm):"=w146:refnum<vi>)
      n95 = Unbundle By Name(w3) -> ("Motion Module.SwaySpeed Set"=w142:refnum<vi>)
      n96 = Unbundle By Name(w3) -> ("Motion Module.Scratch Mode"=w91:refnum<vi>)
      n97 = Unbundle By Name(w3) -> ("Motion Module.HomeScratch"=w86:refnum<vi>)
      n98 = Unbundle By Name(w3) -> ("Motion Module.No of Scratch"=w6:refnum<vi>)
      n99 = Unbundle By Name(w3) -> ("Motion Module.HomeRot"=w83:refnum<vi>)
      n100 = property class="DigNum (strict)"(reference=w6, "Visible"=FALSE) -> (reference out=w7:refnum<vi>, error out=w5:errorcluster)  [unwired: 1 in]
      n101 = property class="Bool (strict)"(reference=w83, "Visible"=FALSE ("Value")) -> (reference out=w81:refnum<vi>, error out=w84:errorcluster)  [unwired: 1 in]
      n102 = property class="Bool (strict)"(reference=w162, "Value"=FALSE) -> (reference out=w160:refnum<vi>, error out=w161:errorcluster)  [unwired: 1 in]
      n103 = property class="Bool (strict)"(reference=w165, "Value"=FALSE) -> (reference out=w167:refnum<vi>, error out=w166:errorcluster)  [unwired: 1 in]
      n104 = property class="Bool (strict)"(reference=w169, "Visible"=FALSE ("Value")) -> (reference out=w171:refnum<vi>, error out=w168:errorcluster)  [unwired: 1 in]
      n105 = property class="Ring (strict)"(reference=w174, "Visible"=FALSE ("Value")) -> (reference out=w172:refnum<vi>, error out=w175:errorcluster)  [unwired: 1 in]
      n106 = property class="Ring (strict)"(reference=w177, "Visible"=FALSE ("Value")) -> (reference out=w179:refnum<vi>, error out=w176:errorcluster)  [unwired: 1 in]
      n107 = property class="TabCtl (strict)"(reference=w181, "Visible"=FALSE ("Value")) -> (reference out=w183:refnum<vi>, error out=w182:errorcluster)  [unwired: 1 in]
      n108 = property class="DigNum (strict)"(reference=w185, "Visible"=FALSE ("Value")) -> (reference out=w187:refnum<vi>, error out=w186:errorcluster)  [unwired: 1 in]
      n109 = property class="Bool (strict)"(reference=w189, "Visible"=FALSE ("Value")) -> (reference out=w191:refnum<vi>, error out=w190:errorcluster)  [unwired: 1 in]
      n110 = property class="Ring (strict)"(reference=w158, "Visible"=FALSE ("Value")) -> (reference out=w153:refnum<vi>, error out=w157:errorcluster)  [unwired: 1 in]
      n111 = property class="DigNum (strict)"(reference=w155, "Visible"=FALSE ("Value")) -> (reference out=w152:refnum<vi>, error out=w154:errorcluster)  [unwired: 1 in]
      n112 = property class="DigNum (strict)"(reference=w150, "Visible"=FALSE ("Value")) -> (reference out=w148:refnum<vi>, error out=w149:errorcluster)  [unwired: 1 in]
      n113 = property class="DigNum (strict)"(reference=w146, "Visible"=FALSE ("Value")) -> (reference out=w144:refnum<vi>, error out=w145:errorcluster)  [unwired: 1 in]
      n114 = property class="Bool (strict)"(reference=w142, "Visible"=FALSE ("Value")) -> (reference out=w140:refnum<vi>, error out=w141:errorcluster)  [unwired: 1 in]
      n115 = property class="Ring (strict)"(reference=w91, "Visible"=FALSE ("Value")) -> (reference out=w89:refnum<vi>, error out=w92:errorcluster)  [unwired: 1 in]
      n116 = property class="Bool (strict)"(reference=w86, "Visible"=FALSE ("Value")) -> (reference out=w88:refnum<vi>, error out=w85:errorcluster)  [unwired: 1 in]
      n117 = Close Reference(reference=w7, error in (no error)=w5) -> ()  [unwired: 1 out]
      n118 = Close Reference(reference=w81, error in (no error)=w84) -> ()  [unwired: 1 out]
      n119 = Close Reference(reference=w160, error in (no error)=w161) -> ()  [unwired: 1 out]
      n120 = Close Reference(reference=w167, error in (no error)=w166) -> ()  [unwired: 1 out]
      n121 = Close Reference(reference=w171, error in (no error)=w168) -> ()  [unwired: 1 out]
      n122 = Close Reference(reference=w172, error in (no error)=w175) -> ()  [unwired: 1 out]
      n123 = Close Reference(reference=w179, error in (no error)=w176) -> ()  [unwired: 1 out]
      n124 = Close Reference(reference=w183, error in (no error)=w182) -> ()  [unwired: 1 out]
      n125 = Close Reference(reference=w187, error in (no error)=w186) -> ()  [unwired: 1 out]
      n126 = Close Reference(reference=w191, error in (no error)=w190) -> ()  [unwired: 1 out]
      n127 = Close Reference(reference=w153, error in (no error)=w157) -> ()  [unwired: 1 out]
      n128 = Close Reference(reference=w152, error in (no error)=w154) -> ()  [unwired: 1 out]
      n129 = Close Reference(reference=w148, error in (no error)=w149) -> ()  [unwired: 1 out]
      n130 = Close Reference(reference=w144, error in (no error)=w145) -> ()  [unwired: 1 out]
      n131 = Close Reference(reference=w140, error in (no error)=w141) -> ()  [unwired: 1 out]
      n132 = Close Reference(reference=w89, error in (no error)=w92) -> ()  [unwired: 1 out]
      n133 = Close Reference(reference=w88, error in (no error)=w85) -> ()  [unwired: 1 out]
      n134 = Unbundle By Name(w3) -> ("Environmental control.High Temp"=w110:refnum<vi>)
      n135 = Unbundle By Name(w3) -> ("Environmental control.Low Temp"=w113:refnum<vi>)
      n136 = Unbundle By Name(w3) -> ("Environmental control.Humidity"=w117:refnum<vi>)
      n137 = Unbundle By Name(w3) -> ("Environmental control.Enter the Stage \nTemperature (°C):"=w122:refnum<vi>)
      n138 = Unbundle By Name(w3) -> ("Environmental control.Enter the Temperature (°C):"=w125:refnum<vi>)
      n139 = Unbundle By Name(w3) -> ("Environmental control.Enter the Humidity (%Rh):"=w129:refnum<vi>)
      n140 = Unbundle By Name(w3) -> ("Environmental control.Stage Temperature"=w133:refnum<vi>)
      n141 = Unbundle By Name(w3) -> ("Environmental control.Sample Temperature"=w137:refnum<vi>)
      n142 = Unbundle By Name(w3) -> ("Main Screen.zNL 2"=w108:refnum<vi>)
      n143 = Unbundle By Name(w3) -> ("Main Screen.Load En"=w104:refnum<vi>)
      n144 = Unbundle By Name(w3) -> ("Main Screen.CZ FF"=w98:refnum<vi>)
      n145 = Unbundle By Name(w3) -> ("Main Screen.zFF"=w95:refnum<vi>)
      n146 = property class="DigNum (strict)"(reference=w122, "Visible"=FALSE ("Value")) -> (reference out=w120:refnum<vi>, error out=w123:errorcluster)  [unwired: 1 in]
      n147 = property class="DigNum (strict)"(reference=w125, "Visible"=FALSE ("Value")) -> (reference out=w127:refnum<vi>, error out=w124:errorcluster)  [unwired: 1 in]
      n148 = property class="DigNum (strict)"(reference=w129, "Visible"=FALSE ("Value")) -> (reference out=w131:refnum<vi>, error out=w130:errorcluster)  [unwired: 1 in]
      n149 = property class="Bool (strict)"(reference=w110, "Value"=FALSE) -> (reference out=w80:refnum<vi>, error out=w109:errorcluster)  [unwired: 1 in]
      n150 = property class="Bool (strict)"(reference=w113, "Value"=FALSE) -> (reference out=w115:refnum<vi>, error out=w114:errorcluster)  [unwired: 1 in]
      n151 = property class="Bool (strict)"(reference=w117, "Value"=FALSE) -> (reference out=w119:refnum<vi>, error out=w116:errorcluster)  [unwired: 1 in]
      n152 = property class="Bool (strict)"(reference=w108, "DisabledEnum"=T2."Enabled" ("Disabled")) -> (reference out=w106:refnum<vi>, error out=w107:errorcluster)  [unwired: 1 in]
      n153 = property class="Bool (strict)"(reference=w104, "DisabledEnum"=T2."Enabled" ("Disabled")) -> (reference out=w102:refnum<vi>, error out=w103:errorcluster)  [unwired: 1 in]
      n154 = property class="Bool (strict)"(reference=w98, "DisabledEnum"=T2."Enabled" ("Disabled")) -> (reference out=w97:refnum<vi>, error out=w99:errorcluster)  [unwired: 1 in]
      n155 = property class="Bool (strict)"(reference=w95, "DisabledEnum"=T2."Enabled" ("Disabled")) -> (reference out=w96:refnum<vi>, error out=w94:errorcluster)  [unwired: 1 in]
      n156 = property class="Arr (strict)"(reference=w133, "Visible"=FALSE ("Value")) -> (reference out=w135:refnum<vi>, error out=w134:errorcluster)  [unwired: 1 in]
      n157 = property class="Arr (strict)"(reference=w137, "Visible"=FALSE ("Value")) -> (reference out=w139:refnum<vi>, error out=w138:errorcluster)  [unwired: 1 in]
      n158 = Close Reference(reference=w80, error in (no error)=w109) -> ()  [unwired: 1 out]
      n159 = Close Reference(reference=w115, error in (no error)=w114) -> ()  [unwired: 1 out]
      n160 = Close Reference(reference=w119, error in (no error)=w116) -> ()  [unwired: 1 out]
      n161 = Close Reference(reference=w120, error in (no error)=w123) -> ()  [unwired: 1 out]
      n162 = Close Reference(reference=w127, error in (no error)=w124) -> ()  [unwired: 1 out]
      n163 = Close Reference(reference=w131, error in (no error)=w130) -> ()  [unwired: 1 out]
      n164 = Close Reference(reference=w135, error in (no error)=w134) -> ()  [unwired: 1 out]
      n165 = Close Reference(reference=w139, error in (no error)=w138) -> ()  [unwired: 1 out]
      n166 = Close Reference(reference=w106, error in (no error)=w107) -> ()  [unwired: 1 out]
      n167 = Close Reference(reference=w102, error in (no error)=w103) -> ()  [unwired: 1 out]
      n168 = Close Reference(reference=w97, error in (no error)=w99) -> ()  [unwired: 1 out]
      n169 = Close Reference(reference=w96, error in (no error)=w94) -> ()  [unwired: 1 out]
      n170 = Unbundle By Name(w3) -> ("Environmental control.Sensors Picked"=w37:refnum<vi>)
      n171 = Unbundle By Name(w3) -> ("Environmental control.Acoustic Emission 3"=w78:refnum<vi>)
      n172 = Unbundle By Name(w3) -> ("Environmental control.ECR"=w74:refnum<vi>)
      n173 = Unbundle By Name(w3) -> ("Environmental control.Temperature (Amb)"=w72:refnum<vi>)
      n174 = Unbundle By Name(w3) -> ("Environmental control.Temperature (Chamber)"=w69:refnum<vi>)
      n175 = Unbundle By Name(w3) -> ("Environmental control.Humidity (Chamber)"=w66:refnum<vi>)
      n176 = Unbundle By Name(w3) -> ("Environmental control.Microphone"=w63:refnum<vi>)
      n177 = Unbundle By Name(w3) -> ("Environmental control.Wear"=w60:refnum<vi>)
      n178 = Unbundle By Name(w3) -> ("Environmental control.Vibration"=w57:refnum<vi>)
      n179 = Unbundle By Name(w3) -> ("Main Screen.Test Trip"=w46:refnum<vi>)
      n180 = Unbundle By Name(w3) -> ("Main Screen.Trip Log"=w42:refnum<vi>)
      n181 = property class="Bool (strict)"(reference=w78, "Value"=FALSE) -> (reference out=w79:refnum<vi>, error out=w77:errorcluster)  [unwired: 1 in]
      n182 = property class="Bool (strict)"(reference=w74, "Value"=FALSE) -> (reference out=w76:refnum<vi>, error out=w75:errorcluster)  [unwired: 1 in]
      n183 = property class="Bool (strict)"(reference=w72, "Value"=FALSE) -> (reference out=w71:refnum<vi>, error out=w73:errorcluster)  [unwired: 1 in]
      n184 = property class="Bool (strict)"(reference=w69, "Value"=FALSE) -> (reference out=w70:refnum<vi>, error out=w68:errorcluster)  [unwired: 1 in]
      n185 = property class="Bool (strict)"(reference=w66, "Value"=FALSE) -> (reference out=w65:refnum<vi>, error out=w67:errorcluster)  [unwired: 1 in]
      n186 = property class="Bool (strict)"(reference=w63, "Value"=FALSE) -> (reference out=w64:refnum<vi>, error out=w62:errorcluster)  [unwired: 1 in]
      n187 = property class="Bool (strict)"(reference=w60, "Value"=FALSE) -> (reference out=w59:refnum<vi>, error out=w61:errorcluster)  [unwired: 1 in]
      n188 = property class="Bool (strict)"(reference=w57, "Value"=FALSE) -> (reference out=w58:refnum<vi>, error out=w56:errorcluster)  [unwired: 1 in]
      n189 = property class="Bool (strict)"(reference=w46, "Value"=FALSE) -> (reference out=w47:refnum<vi>, error out=w45:errorcluster)  [unwired: 1 in]
      n190 = property class="Str"(reference=w42, "Value"="") -> (reference out=w41:refnum<vi>, error out=w43:errorcluster)  [unwired: 1 in]
      n191 = property class="Str"(reference=w37, "Value"="") -> (reference out=w38:refnum<vi>, error out=w36:errorcluster)  [unwired: 1 in]
      n192 = Close Reference(reference=w79, error in (no error)=w77) -> ()  [unwired: 1 out]
      n193 = Close Reference(reference=w76, error in (no error)=w75) -> ()  [unwired: 1 out]
      n194 = Close Reference(reference=w71, error in (no error)=w73) -> ()  [unwired: 1 out]
      n195 = Close Reference(reference=w70, error in (no error)=w68) -> ()  [unwired: 1 out]
      n196 = Close Reference(reference=w65, error in (no error)=w67) -> ()  [unwired: 1 out]
      n197 = Close Reference(reference=w64, error in (no error)=w62) -> ()  [unwired: 1 out]
      n198 = Close Reference(reference=w59, error in (no error)=w61) -> ()  [unwired: 1 out]
      n199 = Close Reference(reference=w58, error in (no error)=w56) -> ()  [unwired: 1 out]
      n200 = Close Reference(reference=w47, error in (no error)=w45) -> ()  [unwired: 1 out]
      n201 = Close Reference(reference=w41, error in (no error)=w43) -> ()  [unwired: 1 out]
      n202 = Close Reference(reference=w38, error in (no error)=w36) -> ()  [unwired: 1 out]
      n203 = Unbundle By Name(w3) -> ("About Screen.Heave and Surge COM Port:"=w34:refnum<vi>)
      n204 = Unbundle By Name(w3) -> ("About Screen.Sway COM Port:"=w31:refnum<vi>)
      n205 = Unbundle By Name(w3) -> ("About Screen.Temp Modbus:"=w28:refnum<vi>)
      n206 = Unbundle By Name(w3) -> ("About Screen.Humidity Port:"=w27:refnum<vi>)
      n207 = Unbundle By Name(w3) -> ("About Screen.Ramp Port:"=w13:refnum<vi>)
      n208 = Unbundle By Name(w3) -> ("About Screen.Password"=w22:refnum<vi>)
      n209 = Unbundle By Name(w3) -> ("About Screen.ECR Port:"=w12:refnum<vi>)
      n210 = property class="VISAName"(reference=w34, "DisabledEnum"=T2."Disabled and Grayed Out" ("Disabled")) -> (reference out=w35:refnum<vi>, error out=w33:errorcluster)  [unwired: 1 in]
      n211 = property class="VISAName"(reference=w31, "DisabledEnum"=T2."Disabled and Grayed Out" ("Disabled")) -> (reference out=w32:refnum<vi>, error out=w30:errorcluster)  [unwired: 1 in]
      n212 = property class="VISAName"(reference=w28, "DisabledEnum"=T2."Disabled and Grayed Out" ("Disabled")) -> (reference out=w16:refnum<vi>, error out=w29:errorcluster)  [unwired: 1 in]
      n213 = property class="VISAName"(reference=w27, "DisabledEnum"=T2."Disabled and Grayed Out" ("Disabled")) -> (reference out=w25:refnum<vi>, error out=w26:errorcluster)  [unwired: 1 in]
      n214 = property class="VISAName"(reference=w13, "DisabledEnum"=T2."Disabled and Grayed Out" ("Disabled")) -> (reference out=w8:refnum<vi>, error out=w14:errorcluster)  [unwired: 1 in]
      n215 = property class="VISAName"(reference=w12, "DisabledEnum"=T2."Disabled and Grayed Out" ("Disabled")) -> (reference out=w9:refnum<vi>, error out=w11:errorcluster)  [unwired: 1 in]
      n216 = property class="Str"(reference=w22, "Visible"=FALSE) -> (reference out=w24:refnum<vi>, error out=w23:errorcluster)  [unwired: 1 in]
      n217 = Close Reference(reference=w35, error in (no error)=w33) -> ()  [unwired: 1 out]
      n218 = Close Reference(reference=w32, error in (no error)=w30) -> ()  [unwired: 1 out]
      n219 = Close Reference(reference=w16, error in (no error)=w29) -> ()  [unwired: 1 out]
      n220 = Close Reference(reference=w25, error in (no error)=w26) -> ()  [unwired: 1 out]
      n221 = Close Reference(reference=w24, error in (no error)=w23) -> ()  [unwired: 1 out]
      n222 = Close Reference(reference=w8, error in (no error)=w14) -> ()  [unwired: 1 out]
      n223 = Close Reference(reference=w9, error in (no error)=w11) -> ()  [unwired: 1 out]
    }
    frame Error {
    }
  }
